vi "SelectObjDir.vi"(0 "reference in":refnum<class "Logger.lvclass">, 11 "error in (no error)":errorcluster) -> (4 "reference out":refnum<class "Logger.lvclass">, 15 "error out":errorcluster)   [LabVIEW 2019]
uses:
  Logger.lvclass
  DatabaseInterface_class/DatabaseInterface.lvclass
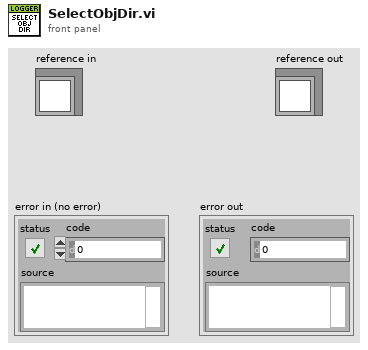
[diagram p1: front panel]
types:
  T1 = typedef "Logger.lvclass/ObjectAttributesRef.ctl" = refnum<data-value>
  T2 = typedef "Logger.lvclass/ObjectAttributes.ctl" = cluster{"queue_event":refnum<queue>, "DatabaseInterface":refnum<class "DatabaseInterface.lvclass">, "queue_device":refnum<queue>}
  T3 = typedef "DatabaseInterface.lvclass/Query Return.ctl" = cluster{"Type of Query":string, "Columns Name":string[], "Columns Data Type":string[], "Row Data":string[][]}
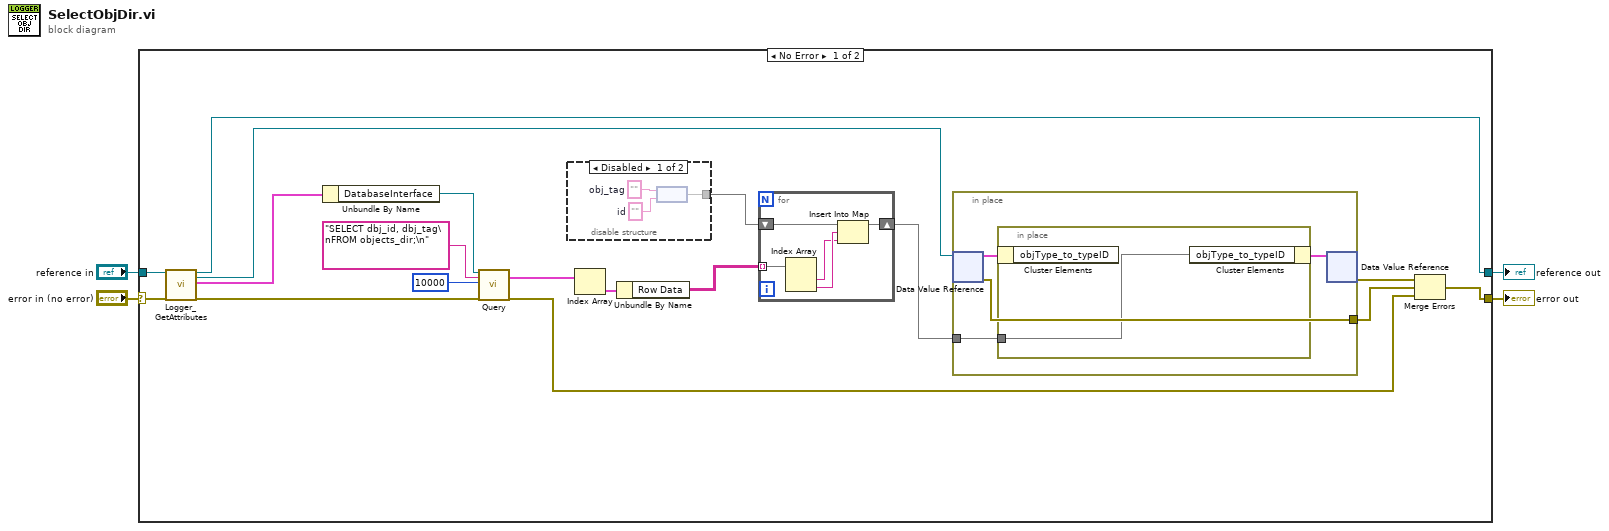
[diagram p0: block diagram]
diagram:
  n1 = case shown="No Error" "error in (no error)" {
    selector: "error in (no error)" -> [w8 w36]
    tunnel: [w22 w36] -> w4
    tunnel: "reference in" -> [w11 w37]
    tunnel: [w7 w37] -> w1
    frame No Error {
      n2 = call "Logger_GetAttributes.vi"("reference in"=w11, "error in (no error)"=w8) -> ("reference out"=w7:refnum<class "Logger.lvclass">, "attributes ref"=w6:T1, "attributes"=w12:T2, "error out"=w9:errorcluster)  [unwired: 14 in]
      n3 = Unbundle By Name(w12) -> ("DatabaseInterface"=w10:refnum<class "DatabaseInterface.lvclass">)
      n4 = call-dynamic "Query.vi"("reference in"=w10, "Query"="SELECT dbj_id, dbj_tag\nFROM objects_dir;\n", "Timeout"=10000, "error in (no error)"=w9) -> ("Query Return"=w19:T3[], "error out"=w5:errorcluster)  [unwired: 13 in, 1 out]
      n5 = disable-structure shown="Disabled" {
        disable-tunnel: [w28 _] -> w17
        frame Disabled {
          w29 = ""  # id
          w30 = ""  # obj_tag
          n6 = node(w30, w29) -> (w28:map{string, string})
        }
        frame Enabled {
        }
      }
      n7 = Index Array(array=w19) -> (element=w15:T3)  [unwired: 1 in]
      n8 = Unbundle By Name(w15) -> ("Row Data"=w16:string[][])
      n9 = for {
        tunnel: w16 -> [w35] mode=indexing
        shift-right: [w33] -> w18
        shift-left: w17 -> [w34]
        n10 = Index Array(array=w35) -> (element #1=w31:string, element #2=w32:string)  [unwired: 2 in]
        n11 = Insert Into Map(map in=w34, key=w32, value=w31) -> (map out=w33:map{string, string})  [unwired: 2 out]
      }
      n12 = in-place {
        in-place-border: w18 -> [w25]
        in-place-border: [w23] -> w21
        n13 = in-place-dvr #1(w6) -> (w26:T2, w23:errorcluster)
        n14 = in-place {
          in-place-border: w25 -> [w27]
          n15 = in-place-cluster #2(w26) -> ()  [unwired: 1 out]
          n16 = in-place-cluster #2("objType_to_typeID"=w27) -> (w24:T2)
        }
        n17 = in-place-dvr #1(w24) -> (w20:errorcluster)  [unwired: 1 out]
      }
      n18 = Merge Errors(w20, w21, w5) -> (w22:errorcluster)
    }
    frame Error {
    }
  }
  "error out" <- w4
  "reference out" <- w1
